vi "data-op.vi"() -> ()   [LabVIEW 2017]
panel:
  out "R4":u8
  in  "A4":u8
  in  "B4":u8
  out "R3":u8
  in  "A3":u8
  in  "B3":u8
  out "R2":u8
  in  "B2":u8
  in  "A2":u8
  out "R1":u8
  in  "B1":u8
  in  "A1":u8
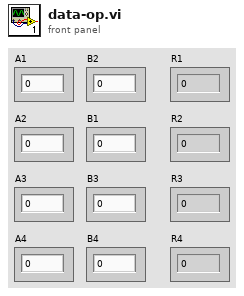
[diagram p1: front panel]
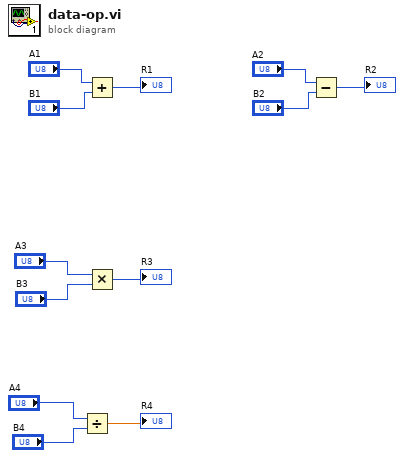
[diagram p0: block diagram]
diagram:
  n1 = Divide(x="A4", y="B4") -> (x/y=→"R4":dbl)
  n2 = Add(x="A1", y="B1") -> (x+y=→"R1":u8)
  n3 = Multiply(x="A3", y="B3") -> (x*y=→"R3":u8)
  n4 = Subtract(x="A2", y="B2") -> (x-y=→"R2":u8)
